vi "getFileLabel.vi"(8 "error in (no error)":errorcluster, 11 "workbook in":refnum<class "workbook.lvclass">) -> (0 "error out":errorcluster, 2 "Default File Label":string, 3 "workbook out":refnum<class "workbook.lvclass">)   [LabVIEW 2017, in "Excel_Specific.lvlib" / "workbook.lvclass"]
uses:
  workbook.lvclass
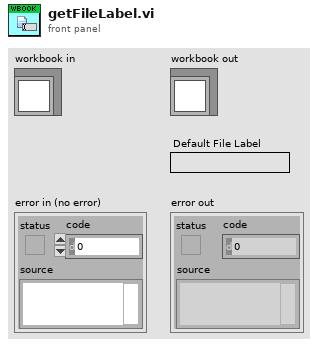
[diagram p1: front panel]
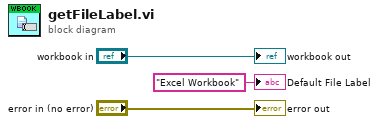
[diagram p0: block diagram]
diagram:
  "error out" <- "error in (no error)"
  "workbook out" <- "workbook in"
  "Default File Label" <- "Excel Workbook" ("Default File Label")
